vi "setup_lc_cz.vi"(0 "zc_luodi_num":string, 1 "fangshi":string, 2 "feiyong":string, 5 "id":string, 9 "yw":string, 12 "syren":string, 14 "shuoming":string) -> (8 "error":errorcluster caption="error out 2")   [LabVIEW 2017, in "Lib_code.lvlib"]
uses:
  Lib_code.lvlib
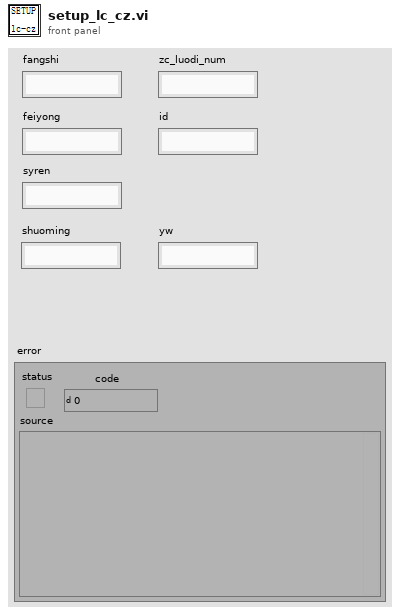
[diagram p1: front panel]
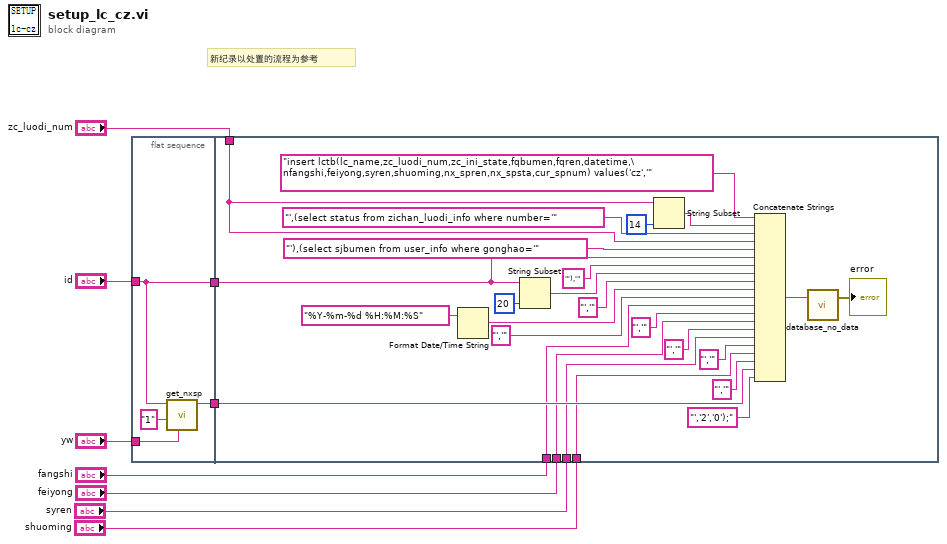
[diagram p0: block diagram]
diagram:
  # "新纪录以处置的流程为参考"
  n1 = flat-sequence {
    tunnel: "id" -> [w12]
    tunnel: [w12] -> w8
    tunnel: [w13] -> w7
    tunnel: "yw" -> [w11]
    tunnel: w8 -> [w29]
    tunnel: w7 -> [w28]
    tunnel: "zc_luodi_num" -> [w25]
    tunnel: "shuoming" -> [w21]
    tunnel: "feiyong" -> [w19]
    tunnel: "fangshi" -> [w16]
    tunnel: "syren" -> [w15]
    frame #0 {
      n2 = call "get_nxsp.vi"("yw"=w11, "Cur_state"="1", "fqren"=w12) -> ("sp_gonghao"=w13:string)  [unwired: 6 in, 2 out]
    }
    frame #1 {
      n3 = Format Date/Time String(time format string (%c)="%Y-%m-%d %H:%M:%S" ("时间格式字符串(%c)")) -> (date/time string=w30:string)  [unwired: 2 in]
      n4 = String Subset(string=w29, length (rest)=20 ("长度（剩余）")) -> (substring=w32:string)  [unwired: 1 in]
      n5 = String Subset(string=w25, length (rest)=14 ("长度（剩余）")) -> (substring=w37:string)  [unwired: 1 in]
      n6 = Concatenate Strings("insert lctb(lc_name,zc_luodi_num,zc_ini_state,fqbumen,fqren,datetime,\nfangshi,feiyong,syren,shuoming,nx_spren,nx_spsta,cur_spnum) values('cz','" ("格式字符串"), w37, "',(select status from zichan_luodi_info where number='" ("字符串"), w25, "'),(select sjbumen from user_info where gonghao='" ("字符串"), w29, "'),'" ("字符串"), w32, "','" ("字符串"), w30, "','" ("字符串"), w16, "','" ("字符串"), w19, "','" ("字符串"), w15, "','" ("字符串"), w21, "','" ("字符串"), w28, "','2','0');" ("字符串")) -> (w23:string)
      n7 = call "database_no_data.vi"("input"=w23) -> ("error"=→"error":errorcluster)  [unwired: 2 in]
    }
  }
